vi "RefNums_Sensors.vi"() -> ()   [LabVIEW 2018]
panel:
  out "Tank Pressure Transducer":string="FrontLeftDrive"
  out "Lower Pressure Transducer":string="FrontLeftDrive"
  out "Front-Left Prox Sensor":string="FrontLeftDrive"
  out "Front-Right Prox Sensor":string="FrontLeftDrive"
  out "Upper Pressure Transducer":string="FrontLeftDrive"
  out "Rear Prox Sensor":string="FrontLeftDrive"
  out "Left Prox Sensor":string="FrontLeftDrive"
  out "Right Prox Sensor":string="FrontLeftDrive"
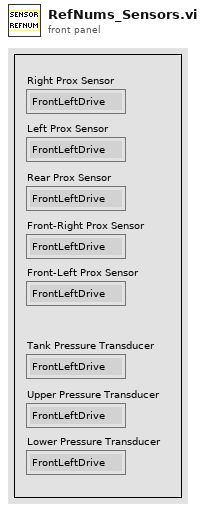
[diagram p1: front panel]
diagram:
